vi "Init Image Gallery.vi"(6 "Shuffle time (5 s)":T1=enum."5s", 7 "Image Gallery in":refnum<class "Image Gallery.lvclass">, 8 "error in (no error)":errorcluster, 9 "Max Size (1024x768)":cluster{"Width":i32, "Height":i32}={"Width"=1024, "Height"=768}, 10 "Path to directory":path, 11 "ImageGallery Title":string) -> (0 "error out":errorcluster, 3 "Image Gallery out":refnum<class "Image Gallery.lvclass">)   [LabVIEW 2012, in "ImageGallery.lvlib" / "Image Gallery.lvclass"]
doc: "Instantiates an object of class \"Image Gallery\".\nThis class is meant to mimic some of the jQuery classes found for javascript."
uses:
  Image Gallery.lvclass
  Shuffle time.ctl
  Image Gallery.lvclass/Image Gallery.ctl
  MessageBox/MessageBox.lvclass
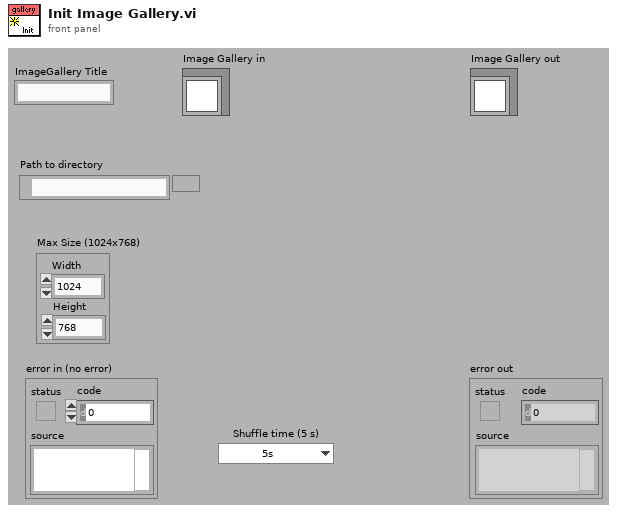
[diagram p1: front panel]
types:
  T1 = typedef "ImageGallery.lvlib/Image Gallery.lvclass/Shuffle time.ctl" = enum16{"Unlimited", "1s", "2s", "3s", "4s", "5s", "7s", "10s", "30s"}
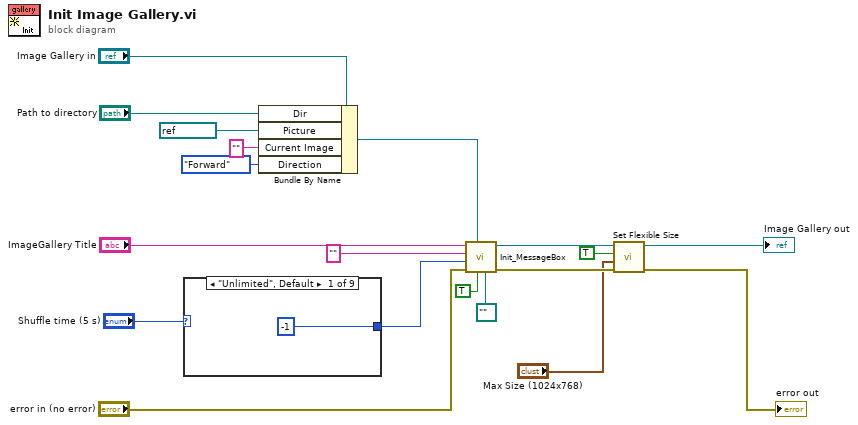
[diagram p0: block diagram]
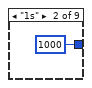
[diagram p2: hidden frame]
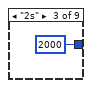
[diagram p3: hidden frame]
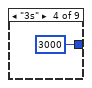
[diagram p4: hidden frame]
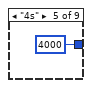
[diagram p5: hidden frame]
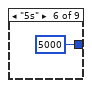
[diagram p6: hidden frame]
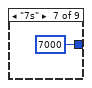
[diagram p7: hidden frame]
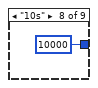
[diagram p8: hidden frame]
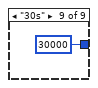
[diagram p9: hidden frame]
diagram:
  n1 = case shown="\"Unlimited\", Default" "Shuffle time (5 s)" {
    tunnel: [-1 ("Timeout (-1)") 1000 ("Timeout (-1)") 2000 ("Timeout (-1)") 3000 ("Timeout (-1)") 4000 ("Timeout (-1)") 5000 ("Timeout (-1)") 7000 ("Timeout (-1)") 10000 ("Timeout (-1)") 30000 ("Timeout (-1)")] -> w10
    frame "Unlimited", Default {
    }
    frame "1s" {
    }
    frame "2s" {
    }
    frame "3s" {
    }
    frame "4s" {
    }
    frame "5s" {
    }
    frame "7s" {
    }
    frame "10s" {
    }
    frame "30s" {
    }
  }
  n2 = Bundle By Name(cluster="Image Gallery in", "Dir"="Path to directory", "Picture"=refnum<vi> refnum, "Current Image"="" ("Message"), "Direction"=enum16{"Forward", "Backward"}."Forward") -> (w17:refnum<class "Image Gallery.lvclass">)
  n3 = call "Init_MessageBox.vi"("Image path"=path "", "Allow to close? (T)"=TRUE, "MessageBox in"=w17, "error in (no error)"="error in (no error)", "Timeout (-1)"=w10, "Message"="", "MsgBox Title"="ImageGallery Title") -> ("error out"=w5:errorcluster, "MessageBox out"=w6:refnum<class "Image Gallery.lvclass">)  [unwired: 3 out]
  n4 = call-dynamic "Set Flexible Size.vi"("error in (no error)"=w5, "Max Size (1024x768)"="Max Size (1024x768)", "Flexible?"=TRUE, "Dialog in"=w6) -> ("error out"=→"error out":errorcluster, "Dialog out"=→"Image Gallery out":refnum<class "Image Gallery.lvclass">)  [unwired: 6 out]
